vi "Generate 1D Motion Profile.vi"(5 "Final Velocity (0)":dbl format="%#_13g", 6 "resolution m (.001)":dbl=0.001 format="%#_13g", 7 "Initial Velocity (0)":dbl format="%#_13g", 8 "Error In":errorcluster, 9 "Max Acceleration":dbl, 10 "Max Velocity":dbl, 11 "Target Position":dbl) -> (0 "Error Out":errorcluster, 3 "Velocity vs Distance Lookup":dbl[](graph))   [LabVIEW 2014, in "Elevator System.lvlib"]
uses:
  Elevator System.lvlib
  <vilib>/Analysis/NI_AALPro.lvlib
panel:
  in  "Initial Position (0)":dbl format="%#_13g"
  out "Perfect Path Following":cluster{"Integral X":dbl[], dbl[]}[](graph)
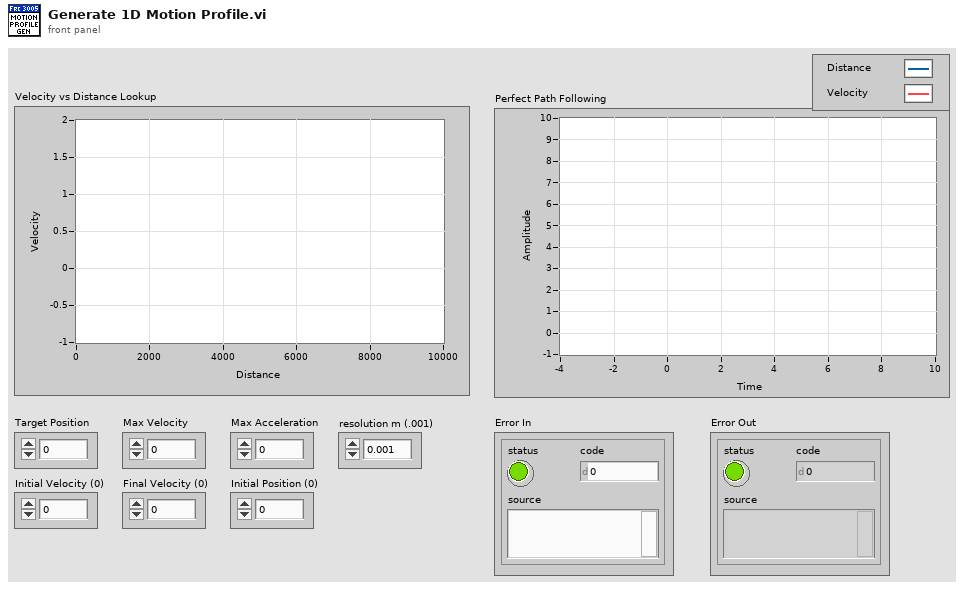
[diagram p1: front panel]
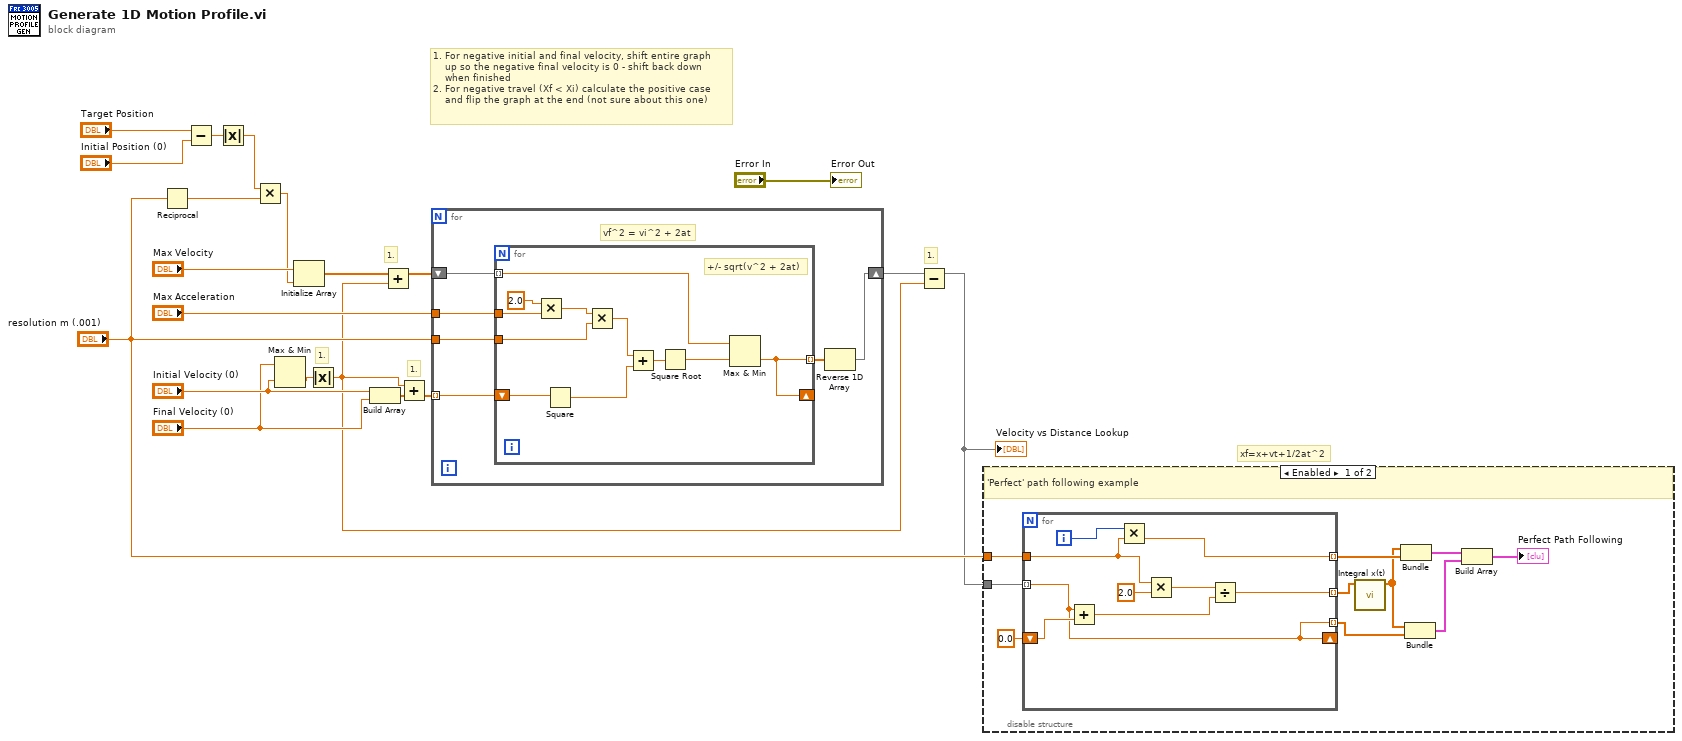
[diagram p0: block diagram]
diagram:
  # "1."
  # "1."
  # "1."
  # "1."
  # "1. For negative initial and final velocity, shift entire graph\n    up so the negative final velocity is 0 - shift back down \n    when finished\n2. For negative travel (Xf < Xi) calculate the positive case\n    and flip the graph at the end (not sure about this one)"
  # "xf=x+vt+1/2at^2"
  n1 = Reciprocal(x="resolution m (.001)") -> (1/x=w20:dbl)
  n2 = Subtract(x="Target Position", y="Initial Position (0)") -> (x-y=w9:dbl)
  n3 = Absolute Value(x=w9) -> (abs(x)=w8:dbl)
  n4 = Multiply(x=w8, y=w20) -> (x*y=w13:dbl)
  n5 = Max & Min(x="Final Velocity (0)", y="Initial Velocity (0)") -> (min(x,y)=w5:dbl)  [unwired: 1 out]
  n6 = Initialize Array("Max Velocity", w13) -> (w14:dbl[])
  n7 = Absolute Value(x=w5) -> (abs(x)=w1:dbl)
  n8 = Build Array("Initial Velocity (0)", "Final Velocity (0)") -> (w12:dbl[])
  n9 = Add(x=w14, y=w1) -> (x+y=w7:dbl[])
  n10 = Add(x=w1, y=w12) -> (x+y=w2:dbl[])
  n11 = for {
    tunnel: "Max Acceleration" -> [w25]
    tunnel: w2 -> [w22] mode=indexing
    tunnel: "resolution m (.001)" -> [w24]
    shift-right: [w26] -> w16
    shift-left: w7 -> [w23]
    # "vf^2 = vi^2 + 2at"
    n12 = for {
      shift-right: [w36] -> _
      shift-left: w22 -> [w28]
      tunnel: [w36] -> w21 mode=indexing
      tunnel: w25 -> [w34]
      tunnel: w23 -> [w37] mode=indexing
      tunnel: w24 -> [w35]
      # "+/- sqrt(v^2 + 2at)"
      n13 = Multiply(x=2.0, y=w34) -> (x*y=w33:dbl)
      n14 = Square(x=w28) -> (x^2=w30:dbl)
      n15 = Multiply(x=w33, y=w35) -> (x*y=w31:dbl)
      n16 = Add(x=w31, y=w30) -> (x+y=w29:dbl)
      n17 = Square Root(x=w29) -> (sqrt(x)=w27:dbl)
      n18 = Max & Min(x=w37, y=w27) -> (min(x,y)=w36:dbl)  [unwired: 1 out]
    }
    n19 = Reverse 1D Array(array=w21) -> (reversed array=w26:dbl[])
  }
  n20 = Subtract(x=w16, y=w1) -> (x-y=w6:dbl[])
  "Velocity vs Distance Lookup" <- w6
  n21 = disable-structure shown="Enabled" {
    disable-tunnel: w6 -> [w47 _]
    disable-tunnel: "resolution m (.001)" -> [w38 _]
    frame Enabled {
      # "'Perfect' path following example"
      n22 = for {
        tunnel: w47 -> [w52] mode=indexing
        shift-right: [w52] -> _
        shift-left: 0.0 -> [w54]
        tunnel: w38 -> [w48]
        tunnel: [w49] -> w44 mode=indexing
        tunnel: [w52] -> w39 mode=indexing
        tunnel: [w50] -> w45 mode=indexing
        i -> [w51]
        n23 = Add(x=w52, y=w54) -> (x+y=w53:dbl)
        n24 = Multiply(x=w51, y=w48) -> (x*y=w49:dbl)
        n25 = Multiply(x=w48, y=2.0) -> (x*y=w55:dbl)
        n26 = Divide(x=w55, y=w53) -> (x/y=w50:dbl)
      }
      n27 = call <vilib>:"Integral x(t).vi"("X"=w45) -> ("Integral X"=w40:dbl[])  [unwired: 9 in, 1 out]
      n28 = Bundle("Integral X"=w40, w44) -> (w42:cluster{"Integral X":dbl[], dbl[]})  [unwired: 1 in]
      n29 = Bundle("Integral X"=w40, w39) -> (w43:cluster{"Integral X":dbl[], dbl[]})  [unwired: 1 in]
      n30 = Build Array(w42, w43) -> (→"Perfect Path Following":cluster{"Integral X":dbl[], dbl[]}[])
    }
    frame Disabled {
    }
  }
  "Error Out" <- "Error In"
